vi "Set Measurement_v1_GetMetadataResponse.vi"(7 "Complete Call (T)":bool=TRUE, 8 "error in (no error)":errorcluster, 10 "Message Data":T1, 11 "gRPCid":T7) -> (0 "error out":errorcluster)   [LabVIEW 2020, in "LineRegulation.lvlib" / "MeasurementService_Template.lvclass"]
uses:
  MeasurementService_Template.lvclass
  <vilib>/gRPC/LabVIEW gRPC Library/Server API/typeDefs/grpcId.ctl
  Measurement_v1_GetMetadataResponse_Data.ctl
  Measurement_v1_MeasurementDetails/Measurement_v1_MeasurementDetails_Data.ctl
  Measurement_v1_MeasurementParameters/Measurement_v1_MeasurementParameters_Data.ctl
  Measurement_v1_ConfigurationParameter/Measurement_v1_ConfigurationParameter_Data.ctl
  Measurement_v1_OutputParameter/Measurement_v1_OutputParameter_Data.ctl
  Measurement_v1_UserInterfaceDetails/Measurement_v1_UserInterfaceDetails_Data.ctl
  dcc74a39-081a-4bdd-860b-8ed792803c96.vi
  <vilib>/gRPC/LabVIEW gRPC Library/Server API/Server/Get Server DLL Path.vi
  <vilib>/Utility/error.llb/Error Cluster From Error Code.vi
  <vilib>/gRPC/LabVIEW gRPC Library/gprc-lvsupport-release.lvlib
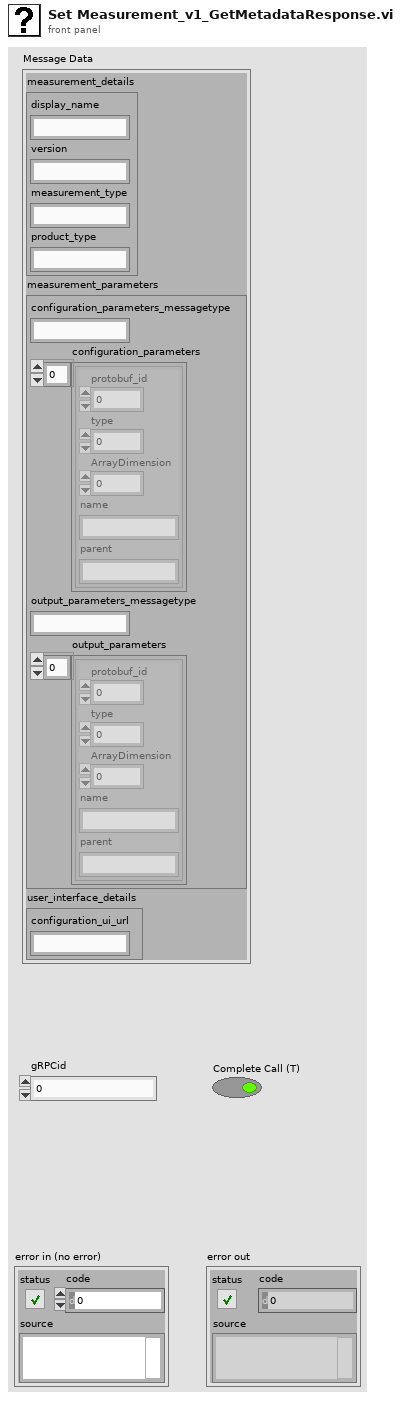
[diagram p1: front panel]
types:
  T1 = typedef "LineRegulation.lvlib/MeasurementService_Template.lvclass/Measurement_v1_GetMetadataResponse_Data.ctl" = cluster{"measurement_details":T2, "measurement_parameters":T3, "user_interface_details":T6}
  T2 = typedef "LineRegulation.lvlib/MeasurementService_Template.lvclass/Measurement_v1_MeasurementDetails_Data.ctl" = cluster{"display_name":string, "version":string, "measurement_type":string, "product_type":string}
  T3 = typedef "LineRegulation.lvlib/MeasurementService_Template.lvclass/Measurement_v1_MeasurementParameters_Data.ctl" = cluster{"configuration_parameters_messagetype":string, "configuration_parameters":T4[], "output_parameters_messagetype":string, "output_parameters":T5[]}
  T4 = typedef "LineRegulation.lvlib/MeasurementService_Template.lvclass/Measurement_v1_ConfigurationParameter_Data.ctl" = cluster{"protobuf_id":i32, "type":i32, "ArrayDimension":i32, "name":string, "parent":string}
  T5 = typedef "LineRegulation.lvlib/MeasurementService_Template.lvclass/Measurement_v1_OutputParameter_Data.ctl" = cluster{"protobuf_id":i32, "type":i32, "ArrayDimension":i32, "name":string, "parent":string}
  T6 = typedef "LineRegulation.lvlib/MeasurementService_Template.lvclass/Measurement_v1_UserInterfaceDetails_Data.ctl" = cluster{"configuration_ui_url":string}
  T7 = typedef "gprc-lvsupport-release.lvlib/grpcId.ctl" = u64
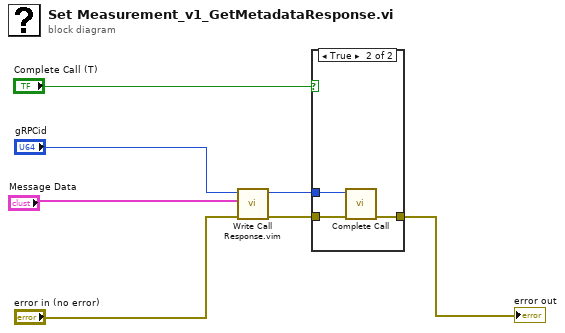
[diagram p0: block diagram]
diagram:
  n1 = call "Write Call Response.vim"("error in (no error)"="error in (no error)", "Response Data"="Message Data", "gRPCid in"="gRPCid") -> ("error out"=w4:errorcluster, "gRPCid"=w5:T7)  [unwired: 7 in]
  n2 = case shown="True" "Complete Call (T)" {
    tunnel: [w8 w11] -> w7
    tunnel: w5 -> [_ w10]
    tunnel: w4 -> [w8 w9]
    frame False {
    }
    frame True {
      n3 = call <vilib>:"Complete Call.vi"("gRPCid"=w10, "error in (no error)"=w9) -> ("error out"=w11:errorcluster)  [unwired: 8 in]
    }
  }
  "error out" <- w7
